vi "SCD41-string-array-to-data.vi"(9 "Starting Index":i32, 11 "Data In (string array)":string[](array[string])) -> (1 "SCD41: Humidity (%)":dbl format="%.2f", 2 "SCD41: Temp (degC)":dbl format="%.2f", 3 "SCD41: CO2 (ppm)":dbl format="%.2f")   [LabVIEW 2021]
panel:
  out "CD1: Humidity":string
  out "SCD41: Temp":string
  out "SCD41: CO2":string
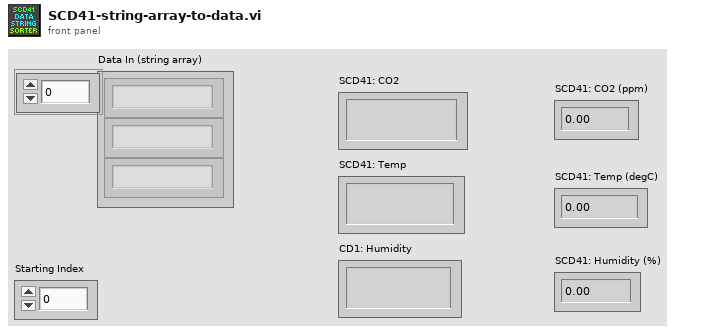
[diagram p1: front panel]
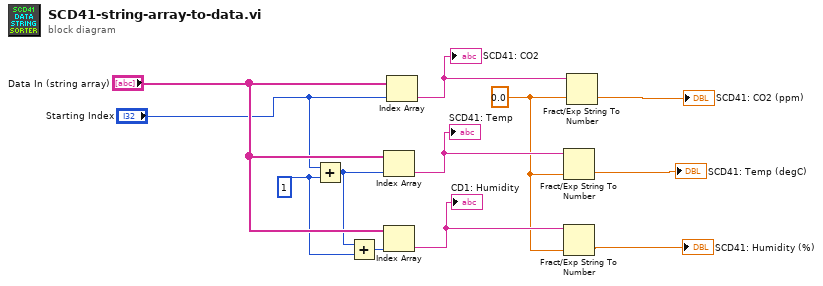
[diagram p0: block diagram]
diagram:
  w8 = 1 ("y")
  w2 = 0.0
  n1 = Add(x="Starting Index", y=w8) -> (x+y=w9:i32)
  n2 = Add(x=w9, y=w8) -> (x+y=w10:i32)
  n3 = Index Array(array="Data In (string array)", index=w9) -> (element=w7:string)
  "SCD41: Temp" <- w7
  n4 = Index Array(array="Data In (string array)", index=w10) -> (element=w3:string)
  "CD1: Humidity" <- w3
  n5 = Index Array "Index Array"(array="Data In (string array)", index="Starting Index") -> (element=w4:string)
  "SCD41: CO2" <- w4
  n6 = Fract/Exp String To Number(string=w7, default (0 dbl)=w2) -> (number=→"SCD41: Temp (degC)":dbl)  [unwired: 2 in, 1 out]
  n7 = Fract/Exp String To Number(string=w3, default (0 dbl)=w2) -> (number=→"SCD41: Humidity (%)":dbl)  [unwired: 2 in, 1 out]
  n8 = Fract/Exp String To Number(string=w4, default (0 dbl)=w2) -> (number=→"SCD41: CO2 (ppm)":dbl)  [unwired: 2 in, 1 out]
